vi "UIRef.vi"(8 "error in":errorcluster, 11 "node in":refnum<class "Target.lvclass">) -> (0 "error out":errorcluster, 2 "VI refnum":refnum<vi>, 3 "node out":refnum<class "Target.lvclass">)   [LabVIEW 2015, in "Target.lvclass"]
doc: "Stores the static reference to the UI of the node."
uses:
  Target.lvclass
  TargetUI.vi
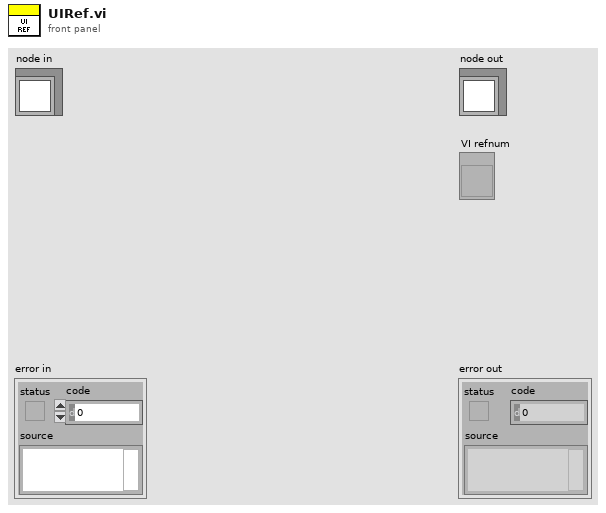
[diagram p1: front panel]
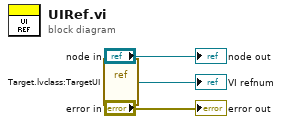
[diagram p0: block diagram]
diagram:
  n1 = vi-ref "Target.lvclass:TargetUI.vi"() -> (→"VI refnum":refnum<vi>)
  "error out" <- "error in"
  "node out" <- "node in"
